vi "pySSHInterface.vi"(4 "Start microPython?":bool=TRUE, 5 "password":string="maker", 6 "Task in":T1(ring)=enum."close", 7 "Username":string="robot", 8 "EOL":string, 10 "Text to write":string="\n\n", 11 "EV3 IP Address":string="192.168.1.36") -> (1 "Init String":string="\n\n", 2 "text read":string="ReadSSH", 3 "Connected?":bool=TRUE)   [LabVIEW 2019]
uses:
  <userlib>/MicroPython/VIs/SSH/PythonVersion.vi
  <vilib>/httpClient/LabVIEWHTTPClient.lvlib
  <vilib>/httpClient/POSTBuffer.vi
panel:
  out "last string":string="ReadSSH"
  in  "IP Address":string
  in  "String to write":string
  out "reply":string
  in  "Task":enum16{"Init", "Read", "Write", "Close"}(ring)
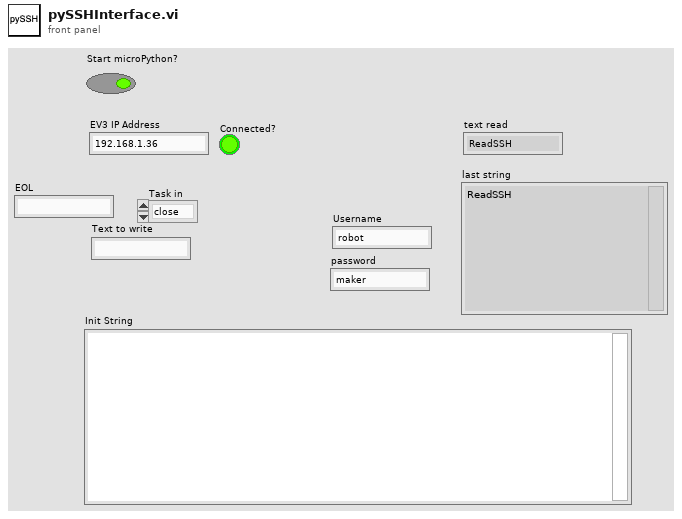
[diagram p1: front panel]
types:
  T1 = enum16{"init", "read", "write", "close", "wait", "reply"}
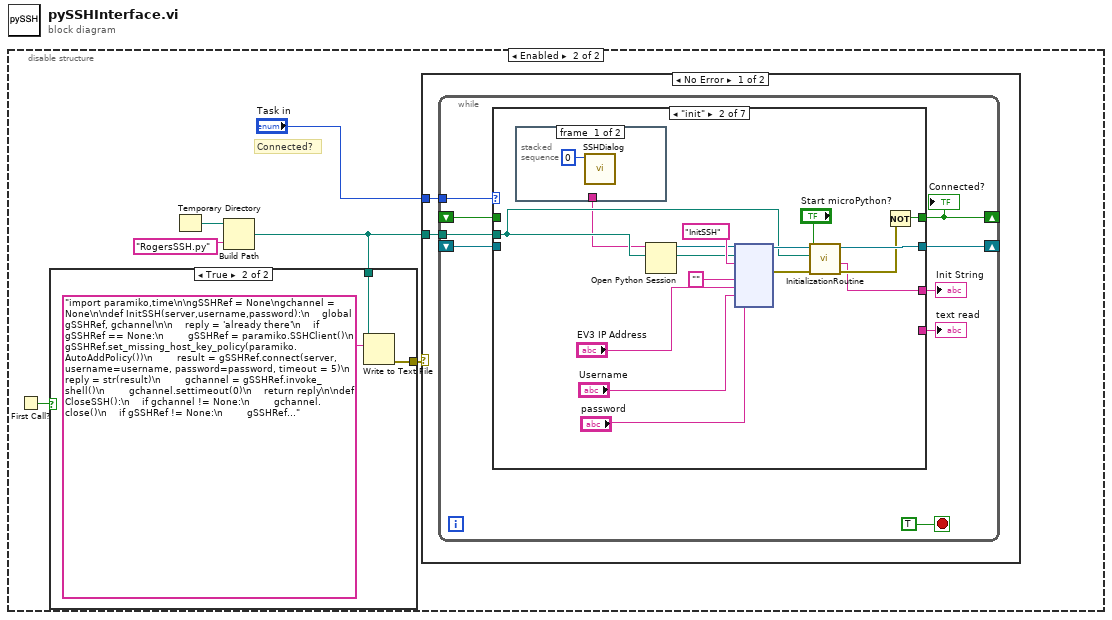
[diagram p0: block diagram]
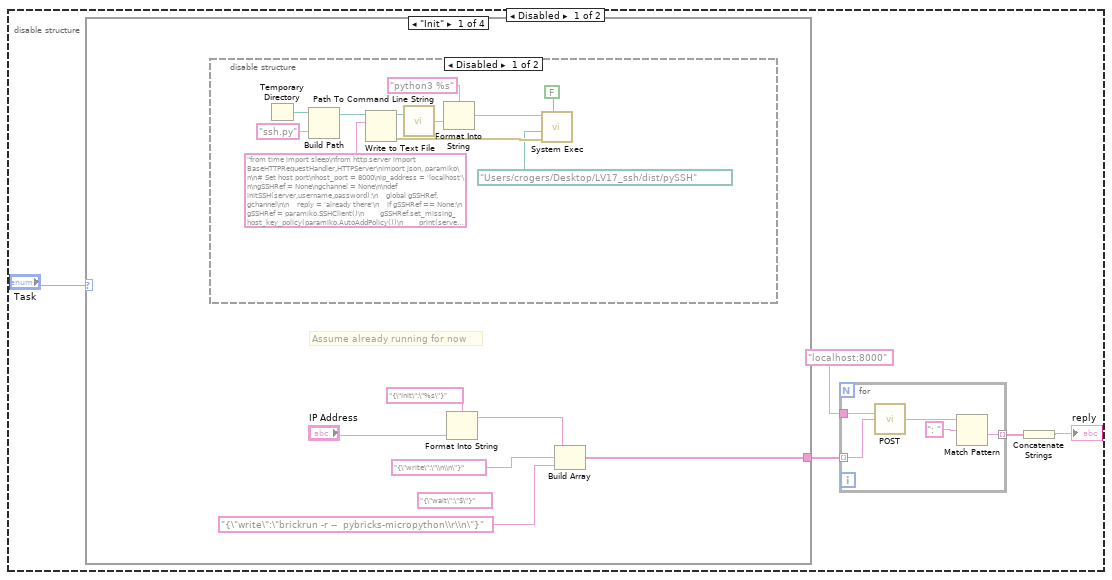
[diagram p2: hidden frame]
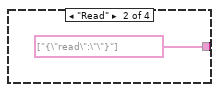
[diagram p4: hidden frame]
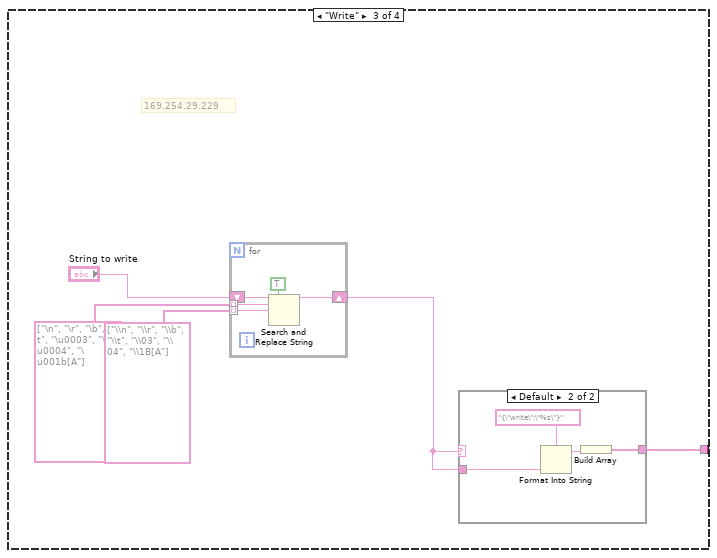
[diagram p5: hidden frame]
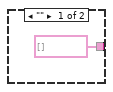
[diagram p6: hidden frame]
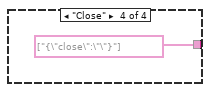
[diagram p7: hidden frame]
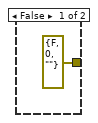
[diagram p8: hidden frame]
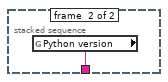
[diagram p10: hidden frame]
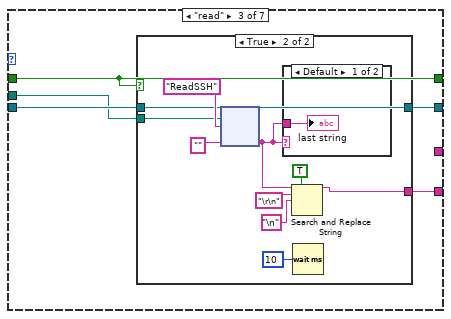
[diagram p11: hidden frame]
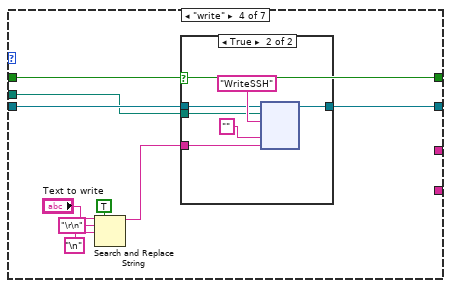
[diagram p14: hidden frame]
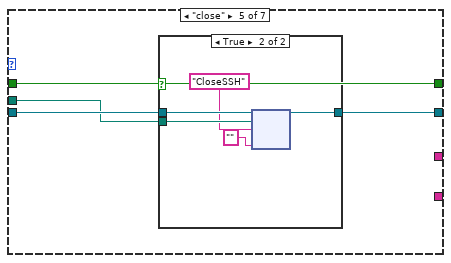
[diagram p16: hidden frame]
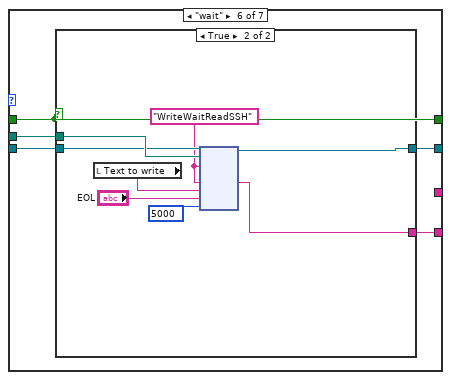
[diagram p18: hidden frame]
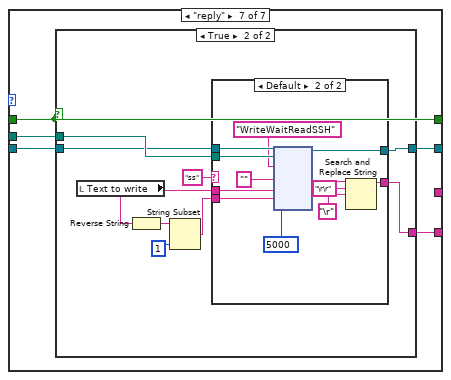
[diagram p20: hidden frame]
diagram:
  n1 = disable-structure shown="Enabled" {
    frame Disabled {
      n2 = case shown="\"Init\"" "Task" {
        tunnel: [w12 string[] ["{\"read\":\"\"}"] ("Array") w32 string[] ["{\"close\":\"\"}"] ("Array")] -> w2
        frame "Init" {
          (unwired) "{\"wait\":\"$\"}" ("buffer")
          # "Assume already running for now"
          n3 = disable-structure shown="Disabled" {
            frame Disabled {
              n4 = Temporary Directory() -> (w26:path)
              n5 = Build Path(base path=w26, name or relative path="ssh.py") -> (appended path=w21:path)
              n6 = Write to Text File(file (use dialog)=w21, text="from time import sleep\nfrom http.server import BaseHTTPRequestHandler,HTTPServer\nimport json, paramiko\n\n# Set host port\nhost_port = 8000\nip_address = 'localhost'\n\ngSSHRef = None\ngchannel = None\n\ndef initSSH(server,username,password):\n    global gSSHRef, gchannel\n\n    reply = 'already there'\n    if gSSHRef == None:\n        gSSHRef = paramiko.SSHClient()\n        gSSHRef.set_missing_host_key_policy(paramiko.AutoAddPolicy())\n        print(server + username + password)\n        result = gSSHRef.connect(server, username=username, password=password, timeout = 5)\n        reply = str(result)\n        gchannel = gSSHRef.invoke_shell()\n        gchannel.settimeout(0)\n    return reply\n\ndef closeSSH():\n    global gSSHRef, gchannel\n    if gchannel != None:\n        gchannel.close()\n    if gSSHRef != None:\n        gSSHRef.close()\n    gSSHRef = None\n    gchannel = None\n    return True\n\ndef writeSSH(string):\n    reply = 'no reference'\n    if gSSHRef != None:\n        reply = 'no file'\n        if gchannel != None:\n            size = gchannel.send(string.encode())\n            reply = str(size)\n    return reply\n\ndef readSSH():\n    reply = 'no reference'\n    if gSSHRef != None:\n        reply = 'no file'\n        if gchannel != None:\n            reply = ''\n            if gchannel.recv_ready():\n                reply = gchannel.recv(9999).decode()\n\n    return(reply)\n\nclass MyServer(BaseHTTPRequestHandler):\n\n    def do_HEAD(self):\n        self.send_response(200)\n        self.send_header('Content-type', 'text/html')\n        self.end_headers()\n\n    def _redirect(self, path):\n        self.send_response(303)\n        self.send_header('Content-type', 'text/html')\n        self.send_header('Location', path)\n        self.end_headers()\n\n    def do_GET(self):\n\n        self.do_HEAD()\n\n    def do_POST(self):\n\n        content_length = int(self.headers['Content-Length'])  # Get the size of data\n        post_data = self.rfile.read(content_length).decode('utf-8')  # Get the data\n        print(post_data)\n        data_array = json.loads(post_data)\n        print(data_array)\n        for data in data_array:\n            print(data)\n            if 'test' in data:\n                print(data['test'])\n                pageContent = 'got: ' + data['test']\n            elif 'init' in data:\n                server = data['init']\n                pageContent = 'init: ' + str(initSSH(server,\"robot\",\"maker\"))\n            elif 'write' in data:\n                pageContent = 'wrote: ' + writeSSH(data['write'])\n            elif 'wait' in data:\n                reply = ''\n                while not data['wait'] in reply:\n                    sleep(1)\n                    reply = reply + readSSH()\n                    print(reply)\n                pageContent = 'wait: ' + reply\n            elif 'read' in data:\n                pageContent = 'read: ' + readSSH()\n            elif 'close' in data:\n                success = closeSSH()\n                pageContent = 'closed' if success else 'failed to close'\n            else:\n                pageCommand = 'Not Supported Command'\n\n        self.wfile.write(pageContent.encode(\"utf-8\"))\n       \n\n# Create Webserver\nif __name__ == '__main__':\n\n    http_server = HTTPServer((ip_address, host_port),MyServer)\n    print(\"Server Starts - %s:%s\" % (ip_address, host_port))\n\n    try:\n        http_server.serve_forever()\n    except KeyboardInterrupt:\n        http_server.server_close()\n        print(\"\\n-------------------EXIT-------------------\")\n\n\n'''\nclass MySSH():\n    def __init(server,username,password):\n        self.server = server\n        self.username = username\n        self.password = password\n        self.gSSHRef = None\n        gchannel = None\n    def init():\n        reply = 'already there'\n        if self.gSSHRef == None:\n            self.gSSHRef = paramiko.SSHClient()\n            self.gSSHRef.set_missing_host_key_policy(paramiko.AutoAddPolicy())\n            result = self.gSSHRef.connect(self.server, self.username, self.password, timeout = 5)\n            reply = str(result)\n            gchannel = self.gSSHRef.invoke_shell()\n            gchannel.settimeout(0)\n        return reply\n    def close():\n        if gchannel != None:\n            gchannel.close()\n        if gSSHRef != None:\n            gSSHRef.close()\n        return True\n    def write(string):\n        reply = 'no reference'\n        if gSSHRef != None:\n            reply = 'no file'\n        if gchannel != None:\n            size = gchannel.send(string.encode())\n            reply = str(size)\n        return reply\n    def read()\n        reply = 'no reference'\n        if gSSHRef != None:\n            reply = 'no file'\n            if gchannel != None:\n                reply = ''\n                if gchannel.recv_ready():\n                    reply = gchannel.recv(9999).decode()\n\n        return(reply)\n        '''\n" ("buffer")) -> (error out=w23:errorcluster)  [unwired: 2 in, 2 out]
              n7 = call <vilib>:"Path To Command Line String.vi"("path"=w21) -> ("string"=w20:string)
              n8 = Format Into String(format string="python3 %s" ("command line"), w20) -> (resulting string=w19:string)  [unwired: 2 in, 1 out]
              n9 = call <vilib>:"System Exec.vi"("wait until completion? (T)"=FALSE, "error in (no error)"=w23, "working directory"=path "/Users/crogers/Desktop/LV17_ssh/dist/pySSH", "command line"=w19) -> ()  [unwired: 4 in, 4 out]
            }
            frame Enabled {
            }
          }
          n10 = Format Into String(format string="{\"init\":\"%s\"}" ("buffer"), "IP Address") -> (resulting string=w14:string)  [unwired: 2 in, 1 out]
          n11 = Build Array(w14, "{\"write\":\"\\n\\n\"}" ("buffer"), "{\"write\":\"brickrun -r --  pybricks-micropython\\r\\n\"}" ("buffer")) -> (w12:string[])
        }
        frame "Read" {
        }
        frame "Write" {
          # "169.254.29.229"
          n12 = for {
            tunnel: string[] ["\n", "\r", "\b", "\t", "\u0003", "\u0004", "\u001b[A"] -> [w34] mode=indexing
            tunnel: string[] ["\\n", "\\r", "\\b", "\\t", "\\03", "\\04", "\\1B[A"] -> [w33] mode=indexing
            shift-right: [w36] -> w28
            shift-left: "String to write" -> [w35]
            n13 = Search and Replace String(replace all?=TRUE ("replace all? (F)"), input string=w35, search string=w34, replace string=w33) -> (result string=w36:string)  [unwired: 4 in, 3 out]
          }
          n14 = case shown="Default" w28 {
            tunnel: w28 -> [_ w42]
            tunnel: [string[] [] w39] -> w32
            frame "" {
            }
            frame Default {
              n15 = Format Into String(format string="{\"write\":\"%s\"}" ("buffer"), w42) -> (resulting string=w40:string)  [unwired: 2 in, 1 out]
              n16 = Build Array(w40) -> (w39:string[])
            }
          }
        }
        frame "Close" {
        }
      }
      n17 = for {
        tunnel: "localhost:8000" ("url") -> [w10]
        tunnel: w2 -> [w9] mode=indexing
        tunnel: [w6] -> w4 mode=indexing
        n18 = call-poly <vilib>:"POST.vi"("url"=w10, "buffer"=w9) -> ("body"=w7:string)  [unwired: 10 in, 3 out]
        n19 = Match Pattern(string=w7, regular expression=": ") -> (after substring=w6:string)  [unwired: 1 in, 3 out]
      }
      n20 = Concatenate Strings(w4) -> (→"reply":string)
    }
    frame Enabled {
      # "Connected?"
      n21 = First Call?() -> (First Call?: T/F=w44:bool)
      n22 = Temporary Directory() -> (w47:path)
      n23 = Build Path(base path=w47, name or relative path="RogersSSH.py") -> (appended path=w48:path)
      n24 = case shown="True" w44 {
        tunnel: [errorcluster {"status"=FALSE, "code"=0, "source"=""} ("error out") w53] -> w49
        tunnel: w48 -> [_ w52]
        frame False {
        }
        frame True {
          n25 = Write to Text File(file (use dialog)=w52, text="import paramiko,time\n\ngSSHRef = None\ngchannel = None\n\ndef InitSSH(server,username,password):\n    global gSSHRef, gchannel\n\n    reply = 'already there'\n    if gSSHRef == None:\n        gSSHRef = paramiko.SSHClient()\n        gSSHRef.set_missing_host_key_policy(paramiko.AutoAddPolicy())\n        result = gSSHRef.connect(server, username=username, password=password, timeout = 5)\n        reply = str(result)\n        gchannel = gSSHRef.invoke_shell()\n        gchannel.settimeout(0)\n    return reply\n\ndef CloseSSH():\n    if gchannel != None:\n        gchannel.close()\n    if gSSHRef != None:\n        gSSHRef.close()\n    return('done')\n\ndef WriteSSH(string):\n    reply = 'no reference'\n    if gSSHRef != None:\n        reply = 'no file'\n        if gchannel != None:\n            size = gchannel.send(string.encode())\n            reply = str(size)\n    return reply\n\ndef ReadSSH():\n    reply = 'no reference'\n    if gSSHRef != None:\n        reply = 'no file'\n        if gchannel != None:\n            reply = ''\n            if gchannel.recv_ready():\n                reply = gchannel.recv(9999).decode()\n\n    return(reply)\n\ndef WriteWaitReadSSH(string,char,timeout=10000):\n     reply =  ReadSSH()\n     WriteSSH(string)\n     n = int(timeout/10)\n     for i in range(n):\n         ans = ReadSSH()\n         if ans.find(char) >= 0:\n             return reply + ans\n         reply = reply + ans\n         time.sleep(0.01)\n     return reply\n\ndef SendLine(string,timeout=10000): # did not work\n     return WriteWaitReadSSH(string,string[-1],timeout)\n\ndef SendSlowly(char,timeout = 2000):\n     reply =  ReadSSH()\n     for char in string:\n          reply = reply + WriteWaitReadSSH(char,char, timeout)\n     return reply\n" ("name or relative path")) -> (error out=w53:errorcluster)  [unwired: 2 in, 2 out]
        }
      }
      n26 = case shown="No Error" w49 {
        tunnel: "Task in" -> [w55 _]
        tunnel: w48 -> [w54 _]
        frame No Error {
          n27 = while {
            shift-right: [w64] -> _
            shift-left: _ -> [w62]
            tunnel: w55 -> [w63]
            tunnel: w54 -> [w61]
            shift-right: [w59] -> _
            shift-left: _ -> [w58]
            stop <- TRUE stop-if-true
            n28 = case shown="\"init\"" w63 {
              tunnel: [w66 w75 w87 w109 w120 w129 w143] -> w64
              tunnel: w62 -> [w66 _ w88 w110 w121 w131 w145]
              tunnel: w61 -> [_ w74 w86 w108 w119 w132 w146]
              tunnel: [w65 w71 w85 w107 w118 w130 w144] -> w59
              tunnel: w58 -> [w65 _ w85 w107 w118 w130 w144]
              tunnel: [_ _ w84 _ _ w128 w142] -> w57
              tunnel: [_ w69 _ _ _ _ _] -> w56
              frame Default {
              }
              frame "init" {
                n29 = stacked-sequence {
                  tunnel: [_ w83] -> w67
                  frame #0 {
                    n30 = call <userlib>:"SSHDialog.vi"("Slide"=u8 0) -> ()  [unwired: 11 in]
                  }
                  frame #1 {
                    n31 = global read "PythonVersion.vi" "Python version"() -> (w83:string)
                  }
                }
                n32 = Open Python Session(python version=w67) -> (session out=w76:refnum<k35>)  [unwired: 2 in, 1 out]
                n33 = node(w76, w74, "InitSSH" ("function name"), "" ("function name"), "EV3 IP Address", "Username", "password") -> (w77:refnum<k35>, w72:errorcluster)  [unwired: 5 in, 2 out]
                n34 = call <userlib>:"InitializationRoutine.vi"("error in (no error)"=w72, "Start microPython?"="Start microPython?", "py file"=w74, "Refnum in"=w77) -> ("error out"=w70:errorcluster, "source"=w69:string, "Refnum out"=w75:refnum<k35>)  [unwired: 5 in]
                n35 = Not(x=w70) -> (.not. x?=w71:bool)
              }
              frame "read" {
                n36 = case shown="True" w85 {
                  tunnel: w88 -> [w89 w99]
                  tunnel: [w89 w98] -> w87
                  tunnel: w86 -> [_ w97]
                  tunnel: [_ w93] -> w84
                  frame False {
                  }
                  frame True {
                    n37 = node(w99, w97, "ReadSSH" ("function name"), "" ("replace string (\"\")")) -> (w98:refnum<k35>, w92:string)  [unwired: 1 in, 3 out]
                    n38 = case shown="Default" w92 {
                      tunnel: w92 -> [w101 _]
                      frame Default {
                        "last string" <- w101
                      }
                      frame "" {
                      }
                    }
                    n39 = Search and Replace String(replace all?=TRUE ("replace all? (F)"), input string=w92, search string="\r\n" ("replace string (\"\")"), replace string="\n" ("replace string (\"\")")) -> (result string=w93:string)  [unwired: 4 in, 3 out]
                    n40 = Wait (ms)(milliseconds to wait=u32 10) -> ()  [unwired: 1 out]
                  }
                }
              }
              frame "write" {
                n41 = Search and Replace String(replace all?=TRUE ("replace all? (F)"), input string="Text to write", search string="\r\n", replace string="\n" ("search string")) -> (result string=w102:string)  [unwired: 4 in, 3 out]
                n42 = case shown="True" w107 {
                  tunnel: w102 -> [_ w117]
                  tunnel: w110 -> [w111 w114]
                  tunnel: [w111 w113] -> w109
                  tunnel: w108 -> [_ w112]
                  frame False {
                  }
                  frame True {
                    n43 = node(w114, w112, "WriteSSH" ("function name"), "" ("function name"), w117) -> (w113:refnum<k35>)  [unwired: 3 in, 3 out]
                  }
                }
              }
              frame "close" {
                n44 = case shown="True" w118 {
                  tunnel: w121 -> [w122 w126]
                  tunnel: [w122 w125] -> w120
                  tunnel: w119 -> [_ w124]
                  frame False {
                  }
                  frame True {
                    n45 = node(w126, w124, "CloseSSH" ("function name"), "" ("function name")) -> (w125:refnum<k35>)  [unwired: 2 in, 3 out]
                  }
                }
              }
              frame "wait" {
                n46 = case shown="True" w130 {
                  tunnel: w132 -> [_ w141]
                  tunnel: w131 -> [w133 w140]
                  tunnel: [w133 w139] -> w129
                  tunnel: [_ w137] -> w128
                  frame False {
                  }
                  frame True {
                    w138 = "WriteWaitReadSSH" ("function name")
                    n47 = local read "Text to write"() -> (w135:string)
                    n48 = node(w140, w141, w138, w138, w135, "EOL", u32 5000 ("milliseconds to wait")) -> (w139:refnum<k35>, w137:string)  [unwired: 4 in, 3 out]
                  }
                }
              }
              frame "reply" {
                n49 = case shown="True" w144 {
                  tunnel: w146 -> [_ w156]
                  tunnel: w145 -> [w147 w155]
                  tunnel: [w147 w154] -> w143
                  tunnel: [_ w153] -> w142
                  frame False {
                  }
                  frame True {
                    n50 = local read "Text to write"() -> (w149:string)
                    n51 = Reverse String(1:w149) -> (0:w152:string)
                    n52 = String Subset(string=w152, length (rest)=1 ("length (rest)")) -> (substring=w150:string)  [unwired: 1 in]
                    n53 = case shown="Default" "ss" {
                      tunnel: w156 -> [_ w170]
                      tunnel: w155 -> [w158 w169]
                      tunnel: [w158 w168] -> w154
                      tunnel: ["" ("function name") w160] -> w153
                      tunnel: w149 -> [_ w165]
                      tunnel: w150 -> [_ w164]
                      frame "" {
                      }
                      frame Default {
                        n54 = node(w169, w170, "WriteWaitReadSSH" ("function name"), "", w165, w164, u32 5000 ("milliseconds to wait")) -> (w168:refnum<k35>, w163:string)  [unwired: 4 in, 3 out]
                        n55 = Search and Replace String(input string=w163, search string="\r\r", replace string="\r" ("search string")) -> (result string=w160:string)  [unwired: 5 in, 3 out]
                      }
                    }
                  }
                }
              }
            }
            "Connected?" <- w59
            "text read" <- w57
            "Init String" <- w56
          }
        }
        frame Error {
          n56 = One Button Dialog(message="Error in saving the python file") -> ()  [unwired: 1 in, 1 out]
        }
      }
    }
  }
